vi "calibrationSpectrometer_monitorCommand_StopImageCapture.vi"(8 "error in (no error)":errorcluster, 11 "command_StopImageCapture_Ctl":T1) -> (0 "error out":errorcluster, 2 "function return":i32, 3 "command_StopImageCapture_Ctl out":T1)   [LabVIEW 2016, in "SALLV_calibrationSpectrometer.lvlib"]
doc: "int calibrationSpectrometer_shm_monitorCommand_StopImageCaptureLV(calibrationSpectrometer_command_StopImageCaptureLV *command_StopImageCapture_Ctl );"
uses:
  SALLV_calibrationSpectrometer.lvlib
  DataTypes/command_StopImageCapture.ctl
  SALLV_calibrationSpectrometer.so
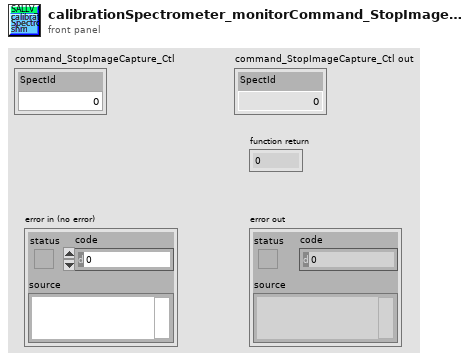
[diagram p1: front panel]
types:
  T1 = typedef "SALLV_calibrationSpectrometer.lvlib/command_StopImageCapture.ctl" = cluster{"SpectId":u16}
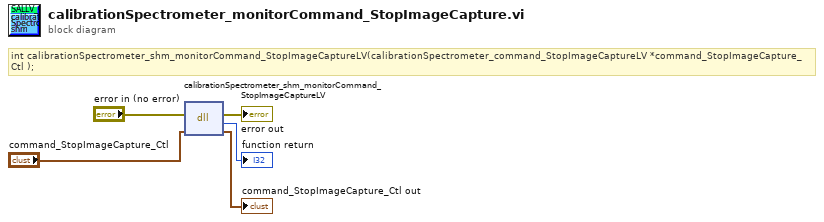
[diagram p0: block diagram]
diagram:
  # "int calibrationSpectrometer_shm_monitorCommand_StopImageCaptureLV(calibrationSpectrometer_command_StopImageCaptureLV *command_StopImageCapture_Ctl );"
  n1 = dll-call lib="home/harini/TCS/sallv_sedspectrometer/SALLV_calibrationSpectrometer.*" fn="calibrationSpectrometer_shm_monitorCommand_StopImageCaptureLV"(error in="error in (no error)", "command_StopImageCapture_Ctl"="command_StopImageCapture_Ctl") -> (error out=→"error out":errorcluster, →"function return":i32, "command_StopImageCapture_Ctl"=→"command_StopImageCapture_Ctl out":T1)  [unwired: 2 in, 1 out]
